vi "簇函数应用.vi"() -> ()   [LabVIEW 2018]
uses:
  <vilib>/Analysis/Matrix/Numeric/Conversions/Array To Matrix - RA.vi
  <vilib>/Analysis/Matrix/NI_Matrix.lvlib
panel:
  in  "簇 3":cluster{"数值":dbl}
  in  "簇 2":cluster{"数值":dbl, "数值 2":dbl, "数值 3":dbl}
  in  "簇":T1
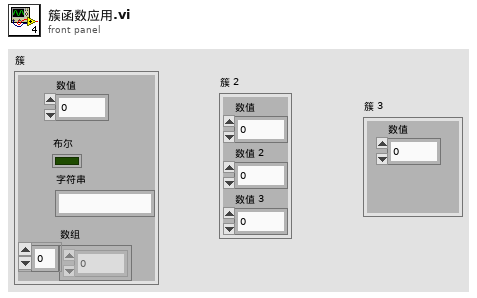
[diagram p1: front panel]
types:
  T1 = cluster{"数值":dbl, "布尔":bool, "字符串":string, "数组":dbl[]}
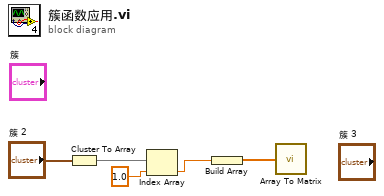
[diagram p0: block diagram]
diagram:
  n1 = Cluster To Array(cluster="簇 2") -> (array=w4:dbl[])
  n2 = Index Array(array=w4, index=1.0 ("元素")) -> (element=w2:dbl)
  n3 = Build Array(w2) -> (w1:dbl[])
  n4 = call-poly <vilib>:"Array To Matrix.vi"("Real 1D Array"=w1) -> ()  [unwired: 1 out]
